vi "NIDCPower_channel_ganging - configure triggers.vi"(8 "error in (no error)":errorcluster, 9 "Measure When":i32(ring)=1025 items=["Automatically after Source Complete"=1025, "On Demand"=1026, "On Measure Trigger"=1027], 11 "Ganged Session In":T1) -> (0 "error out":errorcluster, 3 "Ganged Session Out":T1)   [LabVIEW 2024]
doc: "Automatically configure triggers for Master and Slave sessions for synchronized operation when stacking/ganging"
uses:
  ctl/NIDCPower_channel_ganging - ctl - ganged session.ctl
  ctl/NIDCPower_channel_ganging - ctl - ganged config.ctl
  ctl/NIDCPower_channel_ganging - ctl - channel mode.ctl
  <instrlib>/niDCPower/nidcpower.llb/niDCPower Configure Digital Edge Source Trigger With Channels.vi
  <instrlib>/niDCPower/nidcpower.llb/niDCPower Configure Digital Edge Measure Trigger With Channels.vi
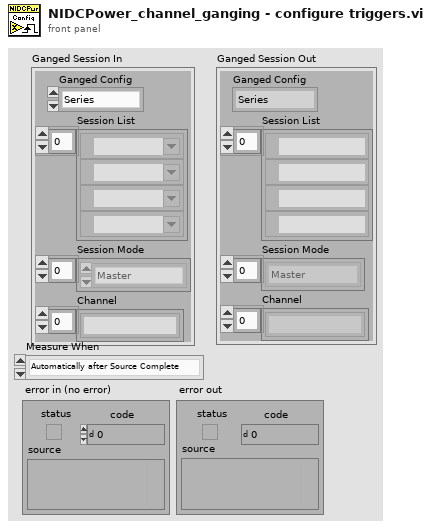
[diagram p1: front panel]
types:
  T1 = typedef "NIDCPower_channel_ganging - ctl - ganged session.ctl" = cluster{"Ganged Config":T2, "Session List":refnum<k15>[], "Session Mode":T3[], "Channel":string[]}
  T2 = typedef "NIDCPower_channel_ganging - ctl - ganged config.ctl" = enum32{"Series", "Parallel", "Manual"}
  T3 = typedef "NIDCPower_channel_ganging - ctl - channel mode.ctl" = enum32{"Master", "Slave", "Slave - Inverted"}
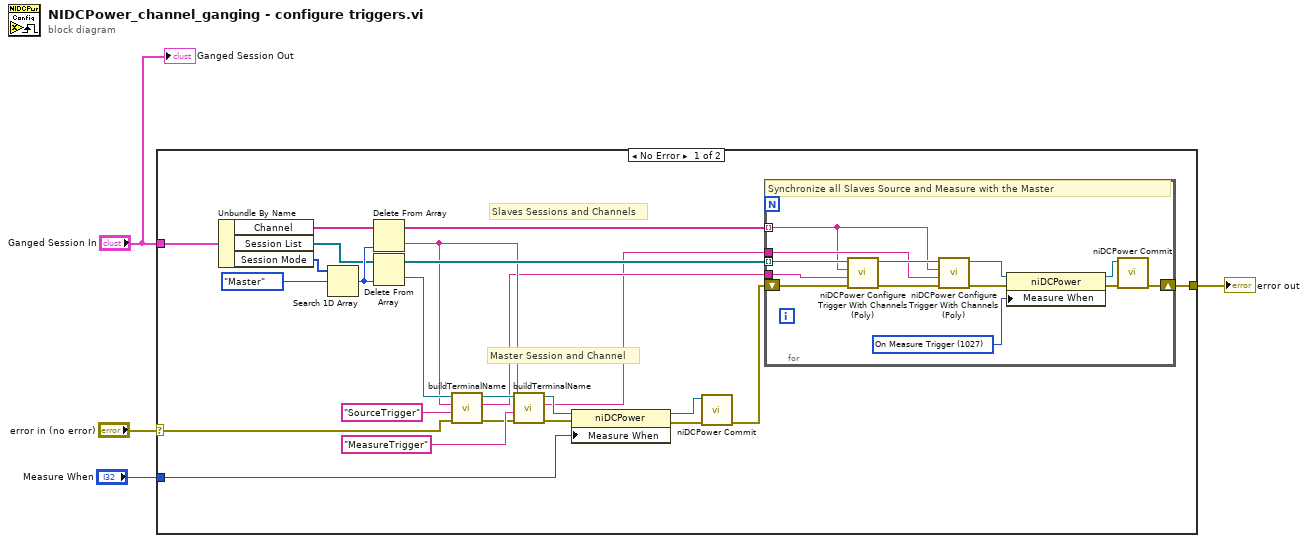
[diagram p0: block diagram]
diagram:
  n1 = case shown="No Error" "error in (no error)" {
    selector: "error in (no error)" -> [w6 w42]
    tunnel: [w28 w42] -> w4
    tunnel: "Ganged Session In" -> [w12 _]
    tunnel: "Measure When" -> [w5 _]
    frame No Error {
      # "Slaves Sessions and Channels"
      # "Master Session and Channel"
      n2 = Unbundle By Name(w12) -> ("Channel"=w25:string[], "Session List"=w24:refnum<k15>[], "Session Mode"=w23:T3[])
      n3 = Search 1D Array(1D array=w23, element=NIDCPower_channel_ganging_-_ctl_-_channel_mode."Master" ("Channel Mode")) -> (index of element=w26:i32)  [unwired: 1 in]
      n4 = Delete From Array(array=w25, index=w26) -> (deleted portion=w11:string, array with subset deleted=w7:string[])  [unwired: 1 in]
      n5 = Delete From Array(array=w24, index=w26) -> (deleted portion=w14:refnum<k15>, array with subset deleted=w15:refnum<k15>[])  [unwired: 1 in]
      n6 = call "buildTerminalName.vi"("error in (no error)"=w6, "Local Terminal Name"="SourceTrigger", "Channel Name"=w11, "session handle"=w14) -> ("error out"=w17:errorcluster, "Fully Qualified Terminal Name"=w10:string, "session handle out"=w16:refnum<k15>)  [unwired: 5 in]
      n7 = call "buildTerminalName.vi"("error in (no error)"=w17, "Local Terminal Name"="MeasureTrigger", "Channel Name"=w11, "session handle"=w16) -> ("error out"=w20:errorcluster, "Fully Qualified Terminal Name"=w9:string, "session handle out"=w19:refnum<k15>)  [unwired: 5 in]
      n8 = property class="niDCPower"(reference=w19, error in=w20, "Measure When"=w5) -> (reference out=w22:refnum<k15>, error out=w21:errorcluster)
      n9 = call <instrlib>:"niDCPower Commit.vi"("error in (no error)"=w21, "instrument handle"=w22) -> ("error out"=w8:errorcluster)  [unwired: 8 in, 1 out]
      n10 = for {
        shift-right: [w40] -> w28
        shift-left: w8 -> [w41]
        tunnel: w15 -> [w39] mode=indexing
        tunnel: w10 -> [w31]
        tunnel: w9 -> [w30]
        tunnel: w7 -> [w29] mode=indexing
        w36 = 1027 items=["Automatically after Source Complete"=1025, "On Demand"=1026, "On Measure Trigger"=1027] ("Measurement:Advanced:Measure When")
        # "Synchronize all Slaves Source and Measure with the Master"
        n11 = call-poly <instrlib>:"niDCPower Configure Trigger With Channels (Poly).vi"("error in (no error)"=w41, "input terminal"=w31, "channel name"=w29, "instrument handle"=w39) -> ("error out"=w38:errorcluster, "instrument handle out"=w37:refnum<k15>)  [unwired: 6 in]
        n12 = call-poly <instrlib>:"niDCPower Configure Trigger With Channels (Poly).vi"("error in (no error)"=w38, "input terminal"=w30, "channel name"=w29, "instrument handle"=w37) -> ("error out"=w35:errorcluster, "instrument handle out"=w34:refnum<k15>)  [unwired: 6 in]
        n13 = property class="niDCPower"(reference=w34, error in=w35, "Measure When"=w36) -> (reference out=w32:refnum<k15>, error out=w33:errorcluster)
        n14 = call <instrlib>:"niDCPower Commit.vi"("error in (no error)"=w33, "instrument handle"=w32) -> ("error out"=w40:errorcluster)  [unwired: 8 in, 1 out]
      }
    }
    frame Error {
    }
  }
  "error out" <- w4
  "Ganged Session Out" <- "Ganged Session In"
